vi "Read_Datalog_Files_110822.vi"() -> ()   [LabVIEW 2011]
uses:
  <vilib>/Utility/file.llb/Read From Spreadsheet File (DBL).vi
panel:
  in  "Numeric 2":dbl
  in  "Numeric":dbl
  out "Waveform Chart 3":dbl[](graph)
  in  "Rápido / Lento":bool
  out "Dias":dbl
  out "Horas":dbl
  out "Total de horas":dbl
  in  "Arquivo de entrada 2":path=path "\\\\Lidar-database\\LIDAR/data/2005/Ago05/0508"
  out "String":string
  out "Array":string[](array[string])
  out "Waveform Chart 2":dbl[](graph)
  out "x = y? 2":bool
  in  "Seleciona Variavel 2":i32
  in  "Seleciona Variavel":i32
  out "all rows":dbl[][](array[numeric]) format="%0.3f"
  out "x = y?":bool
  out "Array size":i32
  # "84    Temperatura\n72    pH\n79    Oxigenio\n67    Dioxido\n80    Pressão\n78    Nivel\n82    Rotação"
  # "C:\\temp\\rotor.lvm"
  # "72, 83, 79, 84, 80, 67, 78"
  # "72, 83, 79, 84, 80, 67, 78"
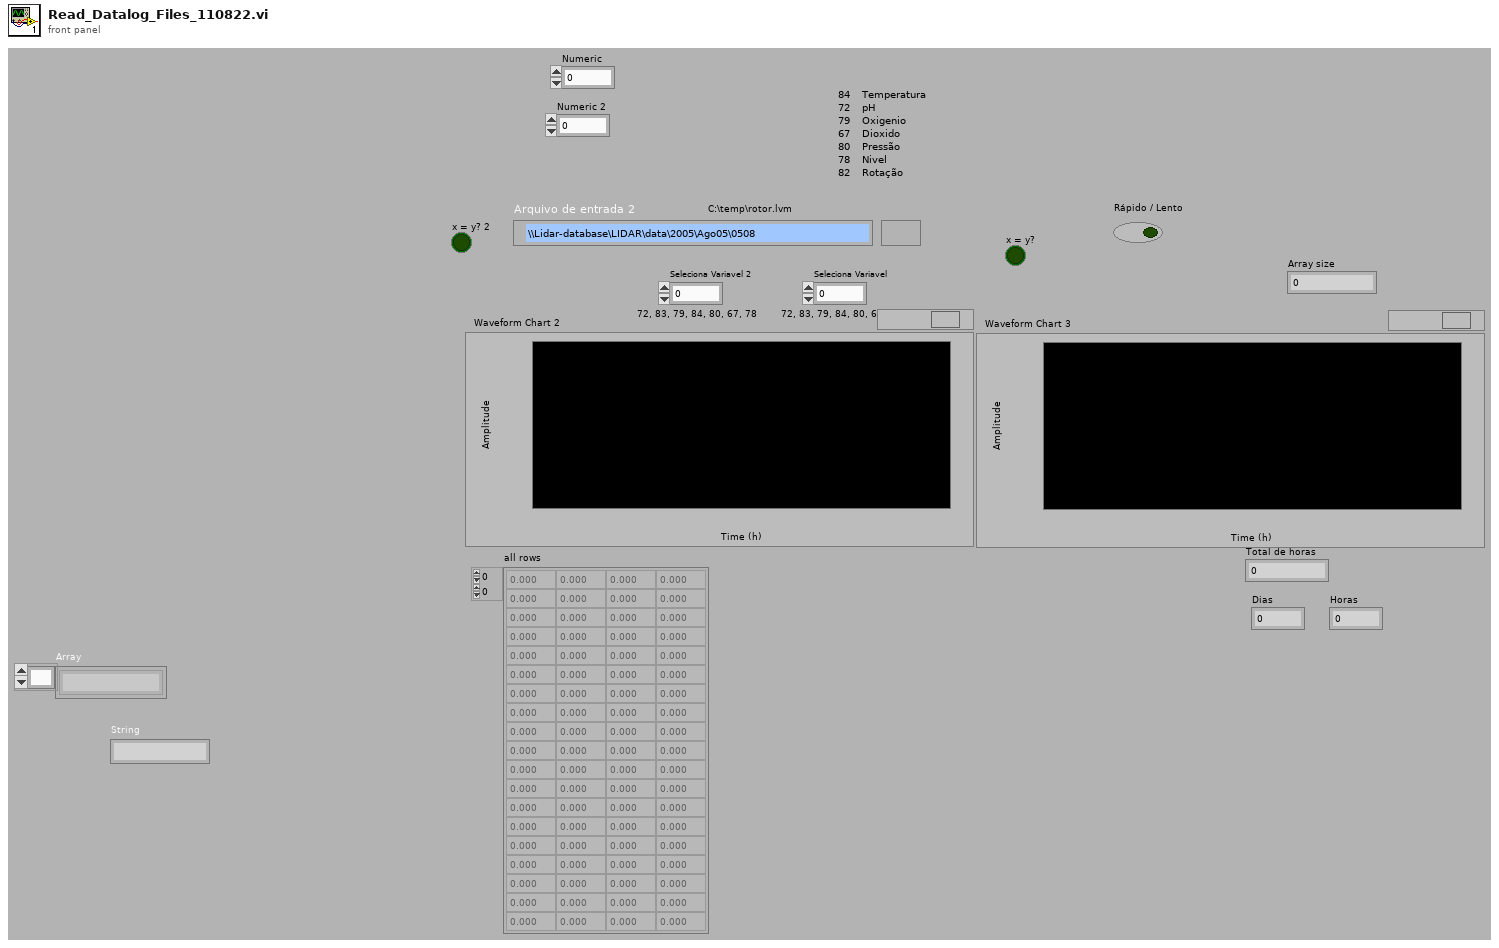
[diagram p1: front panel]
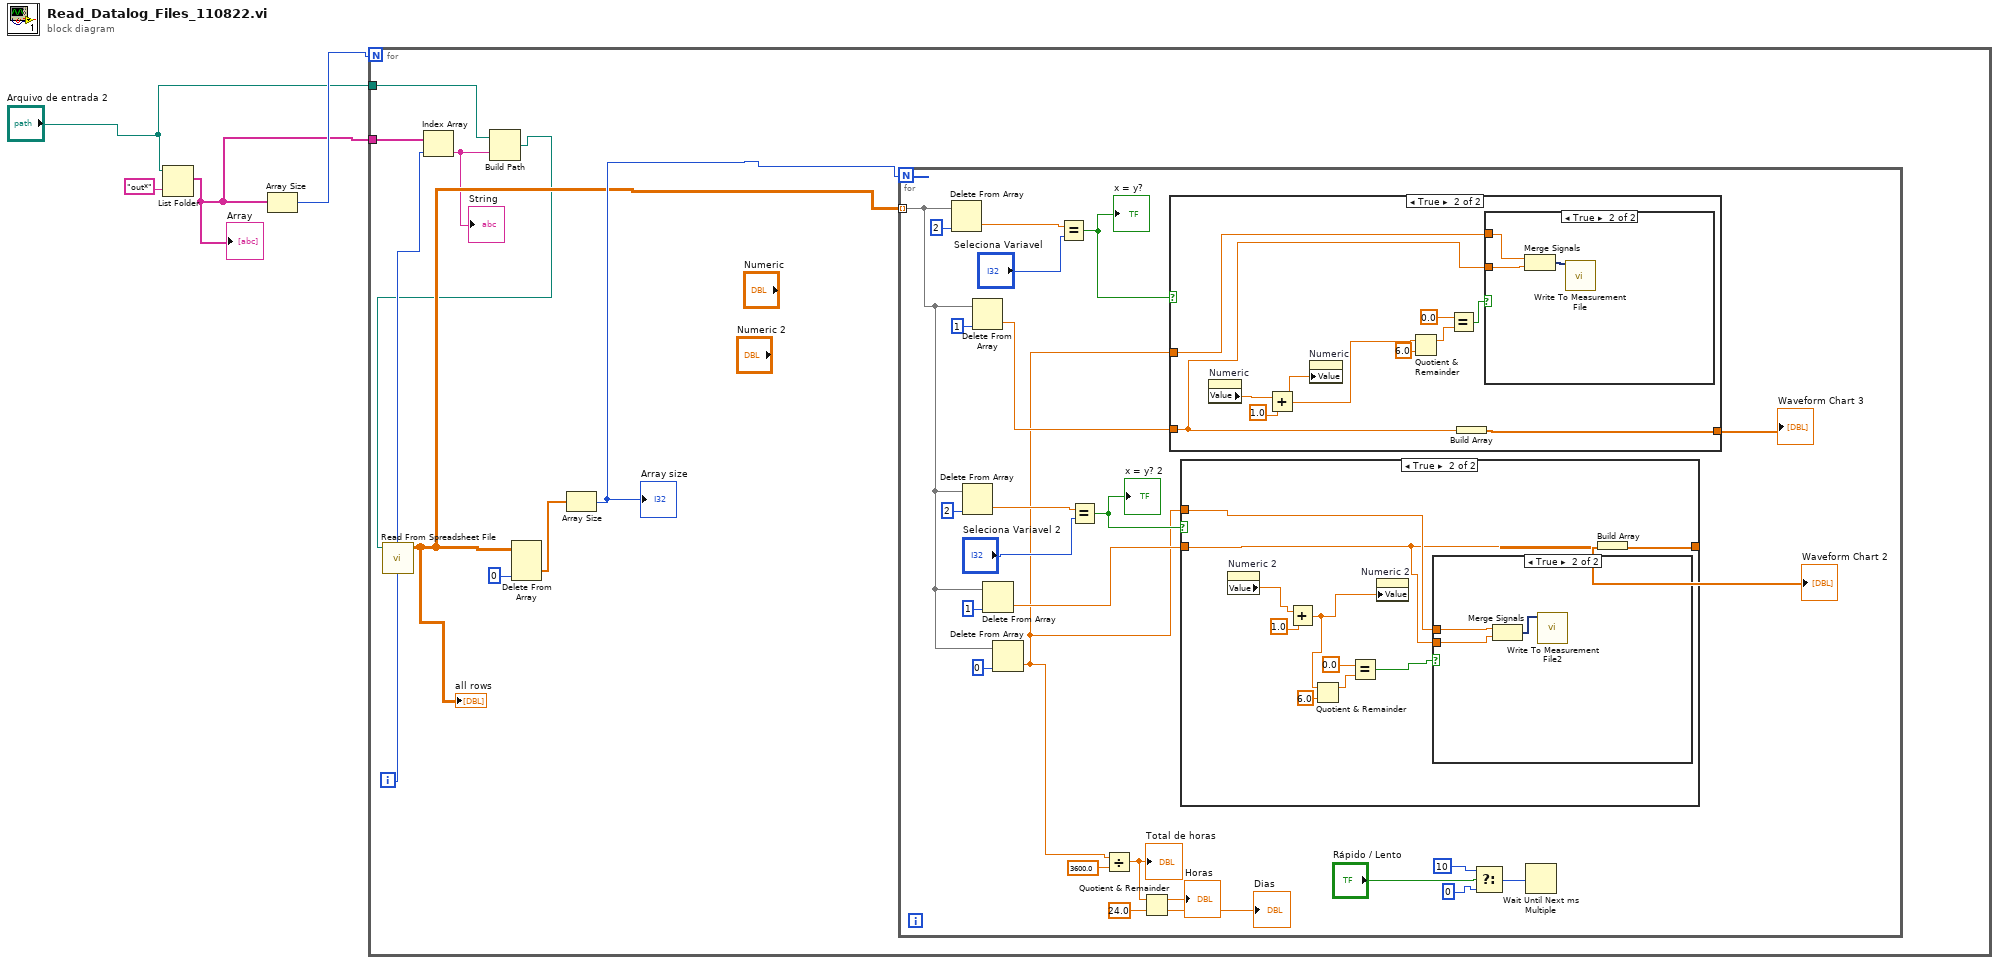
[diagram p0: block diagram]
diagram:
  n1 = List Folder(path="Arquivo de entrada 2", pattern="out*") -> (filenames=w2:string[])  [unwired: 1 in, 4 out]
  "Array" <- w2
  n2 = Array Size(array=w2) -> (size(s)=w3:i32)
  n3 = for {
    N: w3 -> [_]
    tunnel: "Arquivo de entrada 2" -> [w8]
    tunnel: w2 -> [w6]
    i -> [w7]
    n4 = Index Array(array=w6, index=w7) -> (element=w9:string)
    "String" <- w9
    n5 = Build Path(base path=w8, name or relative path=w9) -> (appended path=w5:path)
    n6 = call-poly <vilib>:"Read From Spreadsheet File.vi"("file path (dialog if empty)"=w5) -> ("all rows"=w12:dbl[][])  [unwired: 3 in, 7 out]
    "all rows" <- w12
    n7 = Delete From Array(array=w12, index (col)=0 ("disabled index (row)")) -> (deleted portion=w11:dbl[])  [unwired: 2 in, 1 out]
    n8 = Array Size(array=w11) -> (size(s)=w13:i32)
    "Array size" <- w13
    n9 = for {
      N: w13 -> [_]
      tunnel: w12 -> [w18] mode=indexing
      n10 = Delete From Array(array=w18, index=2) -> (deleted portion=w36:dbl)  [unwired: 1 in, 1 out]
      n11 = Delete From Array(array=w18, index=2) -> (deleted portion=w33:dbl)  [unwired: 1 in, 1 out]
      n12 = Delete From Array(array=w18, index=1) -> (deleted portion=w35:dbl)  [unwired: 1 in, 1 out]
      n13 = Delete From Array(array=w18, index=1) -> (deleted portion=w17:dbl)  [unwired: 1 in, 1 out]
      n14 = Delete From Array(array=w18, index=0) -> (deleted portion=w14:dbl)  [unwired: 1 in, 1 out]
      n15 = Equal?(x=w36, y="Seleciona Variavel") -> (x = y?=w37:bool)
      "x = y?" <- w37
      n16 = Equal?(x=w33, y="Seleciona Variavel 2") -> (x = y?=w32:bool)
      "x = y? 2" <- w32
      n17 = Divide(x=w14, y=3600.0) -> (x/y=w27:dbl)
      "Total de horas" <- w27
      n18 = Quotient & Remainder(x=w27, y=24.0) -> (x-y*floor(x/y)=→"Horas":dbl, floor(x/y)=→"Dias":dbl)
      n19 = case shown="True" w37 {
        tunnel: w35 -> [_ w53]
        tunnel: [_ w62] -> w15
        tunnel: w14 -> [_ w54]
        frame False {
        }
        frame True {
          n20 = property on="Numeric" class="DigNum (strict)"() -> ("Value"=w61:dbl)  [unwired: 2 in, 2 out]
          n21 = Add(x=w61, y=1.0) -> (x+y=w59:dbl)
          n22 = property on="Numeric" class="DigNum (strict)"("Value"=w59) -> ()  [unwired: 2 in, 2 out]
          n23 = Quotient & Remainder(x=w59, y=6.0) -> (x-y*floor(x/y)=w57:dbl)  [unwired: 1 out]
          n24 = Equal?(x=0.0, y=w57) -> (x = y?=w55:bool)
          n25 = Build Array(w53) -> (w62:dbl[])
          n26 = case shown="True" w55 {
            tunnel: w54 -> [_ w64]
            tunnel: w53 -> [_ w63]
            frame False {
            }
            frame True {
              n27 = Merge Signals(w64, w63) -> (w65:dynamicdata)
              n28 = call "Write To Measurement File"("Signals"=w65) -> ()  [unwired: 16 in, 3 out]
            }
          }
        }
      }
      "Waveform Chart 3" <- w15
      n29 = case shown="True" w32 {
        tunnel: w17 -> [_ w41]
        tunnel: [_ w49] -> w16
        tunnel: w14 -> [_ w42]
        frame False {
        }
        frame True {
          n30 = property on="Numeric 2" class="DigNum (strict)"() -> ("Value"=w47:dbl)  [unwired: 2 in, 2 out]
          n31 = Add(x=w47, y=1.0) -> (x+y=w43:dbl)
          n32 = Quotient & Remainder(x=w43, y=6.0) -> (x-y*floor(x/y)=w45:dbl)  [unwired: 1 out]
          n33 = Equal?(x=0.0, y=w45) -> (x = y?=w40:bool)
          n34 = property on="Numeric 2" class="DigNum (strict)"("Value"=w43) -> ()  [unwired: 2 in, 2 out]
          n35 = case shown="True" w40 {
            tunnel: w42 -> [_ w51]
            tunnel: w41 -> [_ w50]
            frame False {
            }
            frame True {
              n36 = Merge Signals(w51, w50) -> (w52:dynamicdata)
              n37 = call "Write To Measurement File2"("Signals"=w52) -> ()  [unwired: 16 in, 3 out]
            }
          }
          n38 = Build Array(w41) -> (w49:dbl[])
        }
      }
      "Waveform Chart 2" <- w16
      n39 = Select(t=u32 10 ("millisecond multiple"), s="Rápido / Lento", f=u32 0 ("millisecond multiple")) -> (s? t:f=w20:u32)
      n40 = Wait Until Next ms Multiple(millisecond multiple=w20) -> ()  [unwired: 1 out]
    }
  }
